vi "Output Error.vi"(8 "error in (no error)":errorcluster) -> (0 "error out":errorcluster)   [LabVIEW 2020, in "neg-pkg-cli.lvlib" / "CLI.lvclass"]
uses:
  CLI.lvclass
  <vilib>/Utility/error.llb/DialogType.ctl
  MGI Console/Source/Console/Console.lvclass
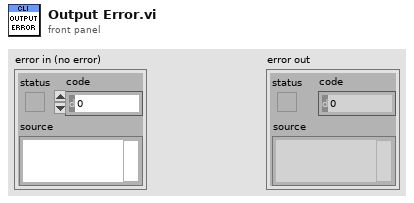
[diagram p1: front panel]
types:
  T1 = typedef "DialogType.ctl" = u16
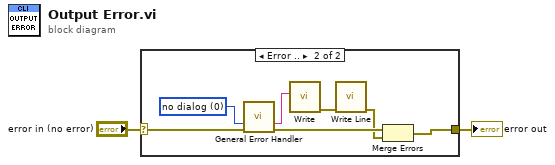
[diagram p0: block diagram]
diagram:
  n1 = case shown="Error .." "error in (no error)" {
    selector: "error in (no error)" -> [w3 w10]
    tunnel: [w3 w4] -> w1
    frame No Error {
    }
    frame Error {
      w9 = T1 0 items=["no dialog", "OK message", "continue or stop message", "OK message + warnings", "continue/stop + warnings"] ("type of dialog (OK msg:1)")
      n2 = call <vilib>:"General Error Handler.vi"("type of dialog (OK msg:1)"=w9, "error in (no error)"=w10) -> ("message"=w8:string, "error out"=w6:errorcluster)  [unwired: 9 in, 3 out]
      n3 = call "Write.vi"("String"=w8) -> ("error out"=w7:errorcluster)  [unwired: 10 in]
      n4 = call "Write Line.vi"("error in (no error)"=w7) -> ("error out"=w5:errorcluster)  [unwired: 10 in]
      n5 = Merge Errors(w6, w5) -> (w4:errorcluster)
    }
  }
  "error out" <- w1
